vi "Get 2D DBL Q on Variant.vi"(8 "error in (no error)":errorcluster, 11 "Variant in":variant) -> (0 "error out":errorcluster, 2 "2D DBL Data Queue":T1, 3 "Variant out":variant)   [LabVIEW 2020, in "Internal Comm Classes.lvlib" / "WPL Comm (2D DBL).lvclass"]
uses:
  WPL Comm (2D DBL).lvclass
  Waveform 2d dbl queue.ctl
  <vilib>/Utility/error.llb/Error Cluster From Error Code.vi
  WPL Comm.lvclass
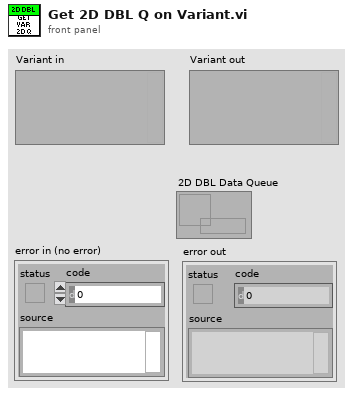
[diagram p1: front panel]
types:
  T1 = typedef "Internal Comm Classes.lvlib/WPL Comm (2D DBL).lvclass/Waveform 2d dbl queue.ctl" = refnum<queue>
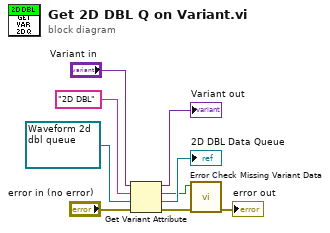
[diagram p0: block diagram]
diagram:
  n1 = Get Variant Attribute(Variant="Variant in", name="2D DBL", default value (empty Variant)=T1 refnum ("2D DBL Data Queue"), error in="error in (no error)") -> (duplicate Variant=→"Variant out":variant, found=w2:bool, value=→"2D DBL Data Queue":T1, error out=w3:errorcluster)
  n2 = call "Error Check Missing Variant Data.vi"("error in (no error)"=w3, "Found?"=w2) -> ("error out"=→"error out":errorcluster)  [unwired: 9 in]
